vi "FetchAllDbl.vi"(8 "error in (no error)":errorcluster, 11 "Simulation in":refnum<class "Simulation.lvclass">) -> (0 "error out":errorcluster, 3 "Simulation out":refnum<class "Simulation.lvclass">)   [LabVIEW 2018, in "DigitizerPlugins.lvlib" / "Simulation.lvclass"]
uses:
  Simulation.lvclass
  F:/Projects/ICDAS/NistPluggableModules/Digitizer/DigitizerPlugins/DigitizerBaseClass/DigitizerBase.lvclass
  DigitizerBaseClass/DigitizerBase.lvclass/DigitizerBase.ctl
  Simulation.lvclass/Simulation.ctl
  DigitizerBaseClass/Typedefs/WfrmAttributes.ctl
  DigitizerBaseClass/Accessors/Read Waveforms.vi
  DigitizerBaseClass/Accessors/Write Waveforms.vi
  Accessors/Read Function.vi
  DigitizerBaseClass/Accessors/Read Acquisition.vi
  DigitizerBaseClass/Accessors/Read Channels.vi
  Accessors/Write Function.vi
  FGen/MemberClasses/FunctionBaseClass/FunctionBase.lvclass
  DigitizerBaseClass/DigitizerBase.lvclass
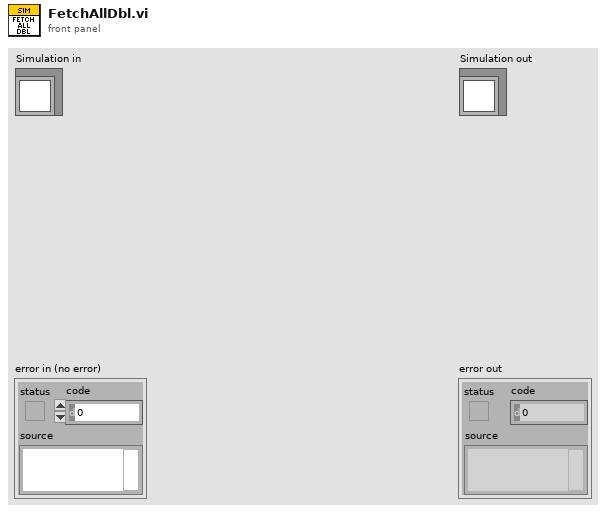
[diagram p1: front panel]
types:
  T1 = typedef "DigitizerPlugins.lvlib/DigitizerBase.lvclass/WfrmAttributes.ctl" = cluster{"XOffset":dbl, "ActualPts":i64, "FirstValid":i64}
  T2 = typedef "DigitizerPlugins.lvlib/DigitizerBase.lvclass/Acquisition.ctl" = cluster{"SampleRate":dbl, "RecordSize":i32, "NumRecords":i32, "SampleMode":i32, "Timeout (ms)":i32}
  T3 = typedef "DigitizerPlugins.lvlib/DigitizerBase.lvclass/Channel.ctl" = cluster{"Name":string, "Enabled":bool, "InputImpedance":dbl, "Coupling":enum16{"AC", "DC", "Gnd"}, "Offset":dbl, "Range":dbl}
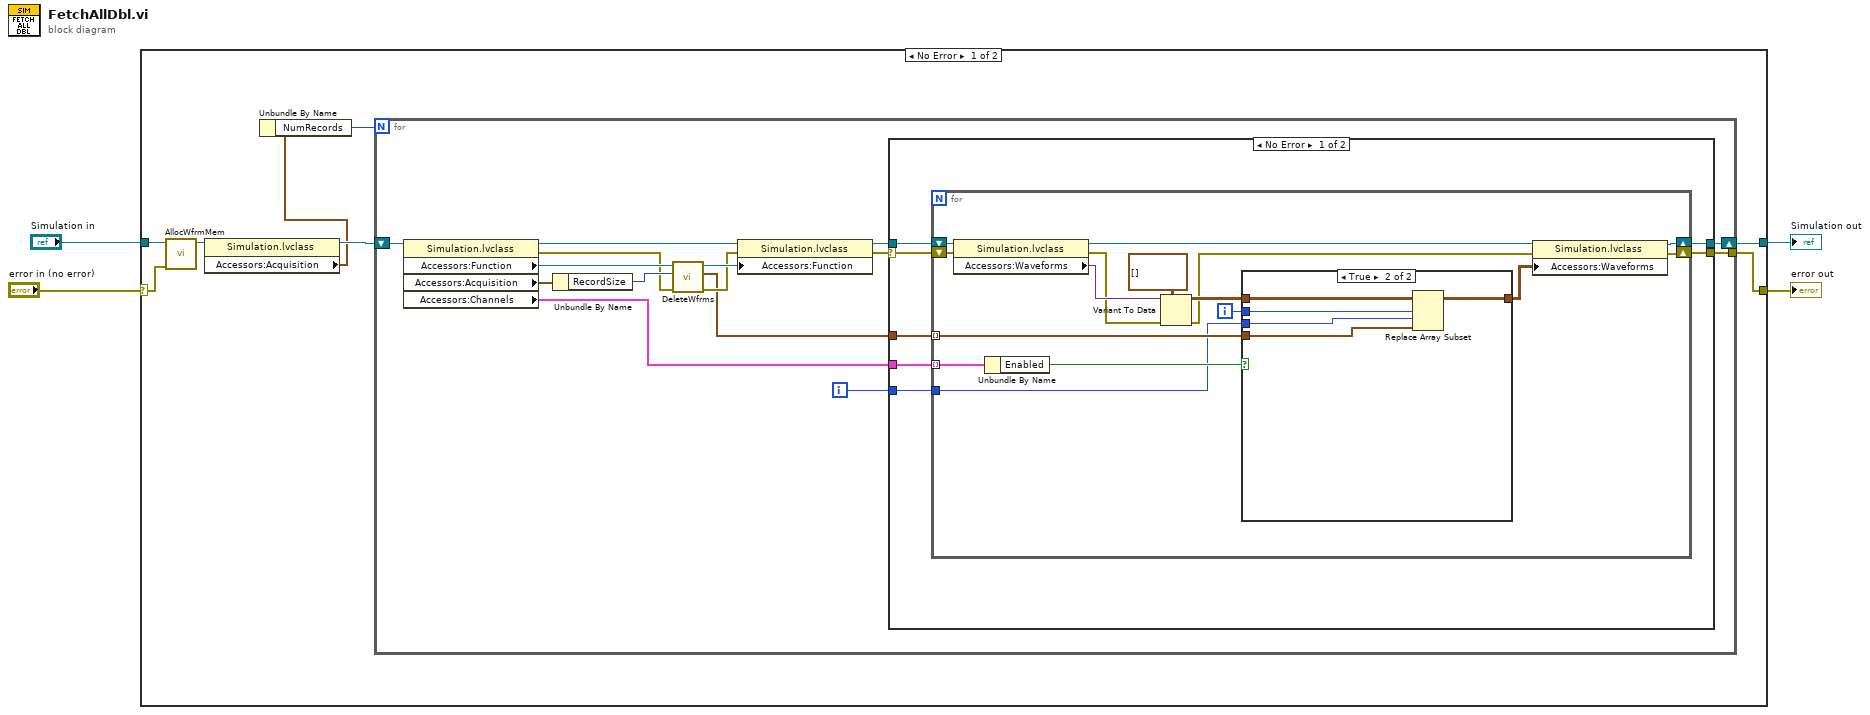
[diagram p0: block diagram]
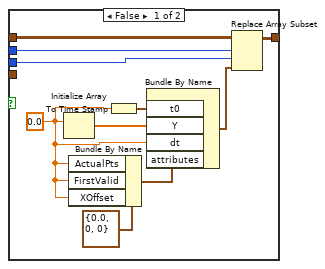
[diagram p2: hidden frame]
diagram:
  n1 = case shown="No Error" "error in (no error)" {
    selector: "error in (no error)" -> [w11 w68]
    tunnel: "Simulation in" -> [w12 w69]
    tunnel: [w9 w69] -> w2
    tunnel: [w8 w68] -> w1
    frame No Error {
      n2 = call-dynamic "AllocWfrmMem.vi"("error in (no error)"=w11, "DigitizerBase in"=w12) -> ("DigitizerBase out"=w10:refnum<class "Simulation.lvclass">)  [unwired: 8 in, 1 out]
      n3 = property class="Simulation.lvclass"(reference=w10) -> (reference out=w7:refnum<class "Simulation.lvclass">, "Accessors:Acquisition"=w6:T2)  [unwired: 1 in, 1 out]
      n4 = Unbundle By Name(w6) -> ("NumRecords"=w5:i32)
      n5 = for {
        N: w5 -> [_]
        tunnel: [w15] -> w8
        shift-right: [w16] -> w9
        shift-left: w7 -> [w14]
        i -> [w13]
        n6 = property class="Simulation.lvclass"(reference=w14) -> (reference out=w27:refnum<class "Simulation.lvclass">, error out=w20:errorcluster, "Accessors:Function"=w22:refnum<class "FunctionBase.lvclass">, "Accessors:Acquisition"=w25:T2, "Accessors:Channels"=w26:T3[])  [unwired: 1 in]
        n7 = Unbundle By Name(w25) -> ("RecordSize"=w21:i32)
        n8 = call "DeleteWfrms.vi"("error in (no error)"=w20, "NumRecords"=w21, "FunctionBase in"=w22) -> ("error out"=w18:errorcluster, "DeletedWaveforms"=w17:waveform(dbl)[], "FunctionBase out"=w19:refnum<class "FunctionBase.lvclass">)  [unwired: 6 in]
        n9 = property class="Simulation.lvclass"(reference=w27, error in=w18, "Accessors:Function"=w19) -> (reference out=w24:refnum<class "Simulation.lvclass">, error out=w23:errorcluster)
        n10 = case shown="No Error" w23 {
          selector: w23 -> [w32 w66]
          tunnel: w26 -> [w34 _]
          tunnel: w24 -> [w33 w67]
          tunnel: w17 -> [w31 _]
          tunnel: [w30 w67] -> w16
          tunnel: [w29 w66] -> w15
          tunnel: w13 -> [w28 _]
          frame No Error {
            n11 = for {
              shift-right: [w41] -> w30
              shift-left: w33 -> [w50]
              shift-right: [w37] -> w29
              shift-left: w32 -> [w49]
              tunnel: w34 -> [w45] mode=indexing
              tunnel: w31 -> [w42] mode=indexing
              tunnel: w28 -> [w35]
              i -> [w36]
              n12 = property class="Simulation.lvclass"(reference=w50, error in=w49) -> (reference out=w39:refnum<class "Simulation.lvclass">, error out=w46:errorcluster, "Accessors:Waveforms"=w47:variant)
              n13 = Unbundle By Name(w45) -> ("Enabled"=w44:bool)
              n14 = Variant To Data(error in=w46, type=waveform(dbl)[][] [], Variant=w47) -> (data=w43:waveform(dbl)[][], error out=w40:errorcluster)
              n15 = case shown="True" w44 {
                tunnel: w43 -> [w53 w65]
                tunnel: w35 -> [w52 w61]
                tunnel: w42 -> [_ w64]
                tunnel: [w54 w63] -> w38
                tunnel: w36 -> [w51 w62]
                frame False {
                  w55 = 0.0 ("element")
                  n16 = Initialize Array(w55) -> (w57:dbl[])  [unwired: 1 in]
                  n17 = Bundle By Name(cluster=T1 {"XOffset"=0.0, "ActualPts"=0, "FirstValid"=0} ("Attributes"), "ActualPts"=w55, "FirstValid"=w55, "XOffset"=w55) -> (w58:T1)
                  n18 = To Time Stamp(1:w55) -> (0:w56:timestamp)
                  n19 = Bundle By Name("t0"=w56, "Y"=w57, "dt"=w55, "attributes"=w58) -> (w60:waveform(dbl))  [unwired: 1 in]
                  n20 = Replace Array Subset(array=w53, new element=w60, index (row)=w51, index (col)=w52) -> (w54:waveform(dbl)[][])
                }
                frame True {
                  n21 = Replace Array Subset(array=w65, new element=w64, index (row)=w62, index (col)=w61) -> (w63:waveform(dbl)[][])
                }
              }
              n22 = property class="Simulation.lvclass"(reference=w39, error in=w40, "Accessors:Waveforms"=w38) -> (reference out=w41:refnum<class "Simulation.lvclass">, error out=w37:errorcluster)
            }
          }
          frame Error {
          }
        }
      }
    }
    frame Error {
    }
  }
  "error out" <- w1
  "Simulation out" <- w2
